vi "LAOnMessage.vi"(8 "Error In":errorcluster, 11 "LiteAgent In":T2) -> (0 "Error Out":errorcluster, 1 "AgentMessage":T1, 2 "SessionId":string, 3 "LiteAgent Out":T2)   [LabVIEW 2017, in "LiteAgentSDK.lvlib"]
uses:
  LiteAgentSDK.lvlib
  C:/Users/Jan/Projects/LiteAgentSDK-LabVIEW/Source/Bin/LiteAgentSDK.LabVIEW.dll
  Bin/LiteAgentSDK.LabVIEW.dll
  <vilib>/LVH/i3 JSON/JSON Parsing/Get Object Parameter Files/Get Object Parameter - String.vi
  <vilib>/LVH/i3 JSON/JSON Parsing/Get Object Parameter Files/Get Object Parameter - Object.vi
  <vilib>/LVH/i3 JSON/i3-json.lvlib
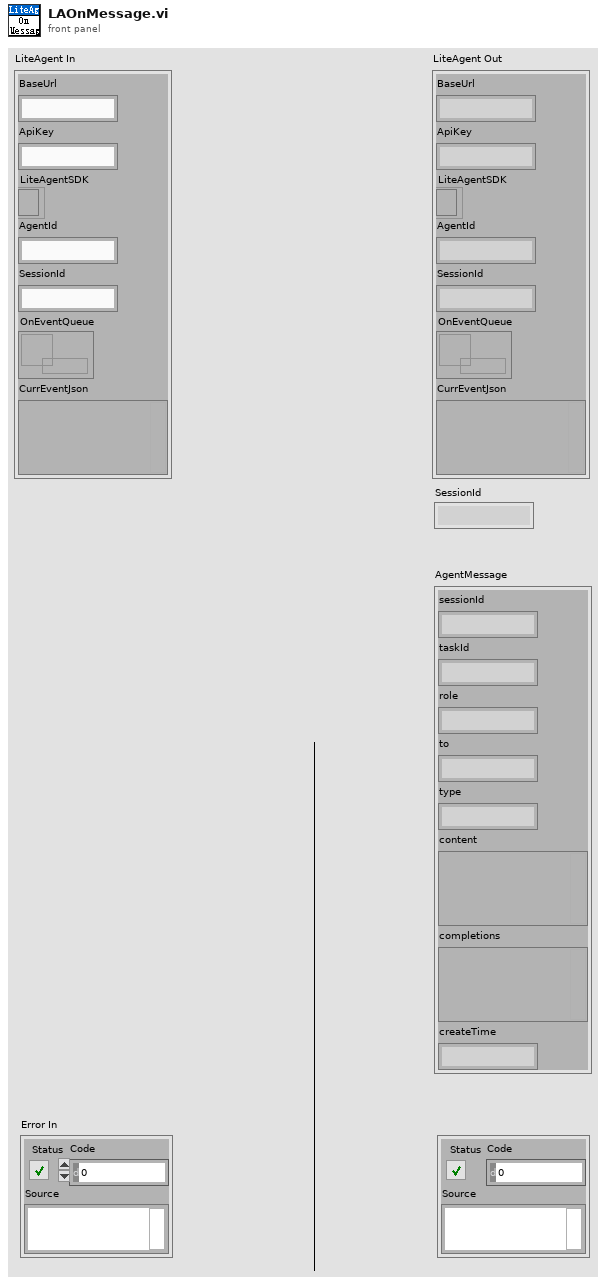
[diagram p1: front panel]
types:
  T1 = cluster{"sessionId":string, "taskId":string, "role":string, "to":string, "type":string, "content":variant, "completions":variant, "createTime":string}
  T2 = cluster{"BaseUrl":string, "ApiKey":string, "LiteAgentSDK":refnum<k24>, "AgentId":string, "SessionId":string, "OnEventQueue":refnum<queue>, "CurrEventJson":variant}
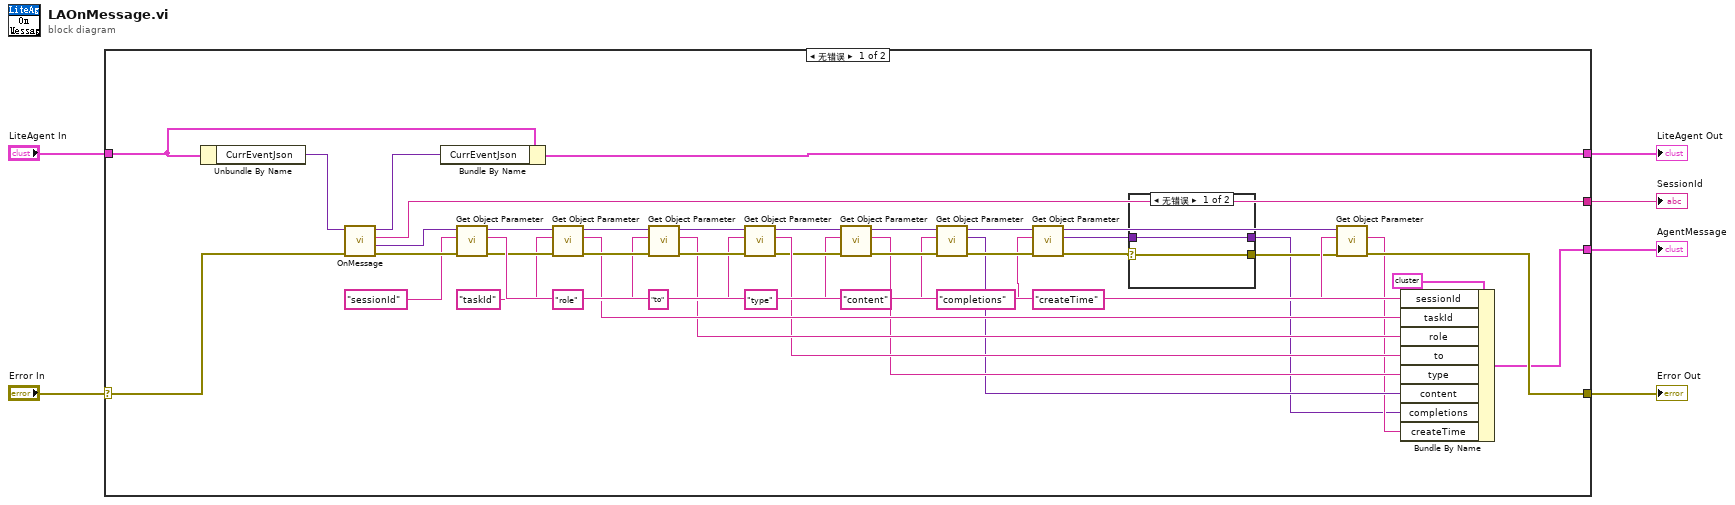
[diagram p0: block diagram]
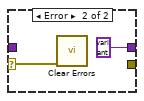
[diagram p2: hidden frame]
diagram:
  n1 = case shown="无错误" "Error In" {
    selector: "Error In" -> [w49 w55]
    tunnel: [w19 w55] -> w5
    tunnel: "LiteAgent In" -> [w47 w54]
    tunnel: [w45 w54] -> w3
    tunnel: [w44 _] -> w2
    tunnel: [w11 _] -> w1
    frame No Error {
      n2 = Unbundle By Name(w47) -> ("CurrEventJson"=w48:variant)
      n3 = call "OnMessage.vi"("Error In"=w49, "JSON Tree In"=w48) -> ("Error Out"=w41:errorcluster, "Payload"=w42:variant, "SessionId"=w44:string, "JSON Tree Out"=w46:variant)  [unwired: 6 in]
      n4 = Bundle By Name(cluster=w47, "CurrEventJson"=w46) -> (w45:T2)
      n5 = call-poly <vilib>:"Get Object Parameter.vi"("error in (no error)"=w41, "Parameter Name"="sessionId", "JSON Tree In (JSON Object)"=w42) -> ("error out"=w37:errorcluster, "String Value"=w39:string, "JSON Tree Out Passthrough"=w38:variant)  [unwired: 5 in, 1 out]
      n6 = call-poly <vilib>:"Get Object Parameter.vi"("error in (no error)"=w37, "Parameter Name"="taskId", "JSON Tree In (JSON Object)"=w38) -> ("error out"=w34:errorcluster, "String Value"=w29:string, "JSON Tree Out Passthrough"=w36:variant)  [unwired: 5 in, 1 out]
      n7 = call-poly <vilib>:"Get Object Parameter.vi"("error in (no error)"=w34, "Parameter Name"="role", "JSON Tree In (JSON Object)"=w36) -> ("error out"=w33:errorcluster, "String Value"=w28:string, "JSON Tree Out Passthrough"=w35:variant)  [unwired: 5 in, 1 out]
      n8 = call-poly <vilib>:"Get Object Parameter.vi"("error in (no error)"=w33, "Parameter Name"="to", "JSON Tree In (JSON Object)"=w35) -> ("error out"=w22:errorcluster, "String Value"=w27:string, "JSON Tree Out Passthrough"=w26:variant)  [unwired: 5 in, 1 out]
      n9 = call-poly <vilib>:"Get Object Parameter.vi"("error in (no error)"=w22, "Parameter Name"="type", "JSON Tree In (JSON Object)"=w26) -> ("error out"=w21:errorcluster, "String Value"=w14:string, "JSON Tree Out Passthrough"=w25:variant)  [unwired: 5 in, 1 out]
      n10 = call-poly <vilib>:"Get Object Parameter.vi"("error in (no error)"=w21, "Parameter Name"="content", "JSON Tree In (JSON Object)"=w25) -> ("error out"=w20:errorcluster, "JSON Object"=w13:variant, "JSON Tree Out Passthrough"=w24:variant)  [unwired: 5 in, 1 out]
      n11 = call-poly <vilib>:"Get Object Parameter.vi"("error in (no error)"=w20, "Parameter Name"="completions", "JSON Tree In (JSON Object)"=w24) -> ("error out"=w10:errorcluster, "JSON Object"=w8:variant, "JSON Tree Out Passthrough"=w23:variant)  [unwired: 5 in, 1 out]
      n12 = case shown="无错误" w10 {
        selector: w10 -> [w51 w53]
        tunnel: [w51 _] -> w9
        tunnel: w8 -> [w50 _]
        tunnel: [w50 variant ("JSON Object")] -> w7
        frame No Error {
        }
        frame Error {
          n13 = call <vilib>:"Clear Errors.vi"("error in (no error)"=w53) -> ()  [unwired: 5 in, 2 out]
        }
      }
      n14 = call-poly <vilib>:"Get Object Parameter.vi"("error in (no error)"=w9, "Parameter Name"="createTime", "JSON Tree In (JSON Object)"=w23) -> ("error out"=w19:errorcluster, "String Value"=w12:string)  [unwired: 5 in, 2 out]
      n15 = Bundle By Name(cluster=T1 {"sessionId"="", "taskId"="", "role"="", "to"="", "type"="", "content"=variant, "completions"=variant, "createTime"=""} ("AgentMessage"), "sessionId"=w39, "taskId"=w29, "role"=w28, "to"=w27, "type"=w14, "content"=w13, "completions"=w7, "createTime"=w12) -> (w11:T1)
    }
    frame Error {
    }
  }
  "Error Out" <- w5
  "LiteAgent Out" <- w3
  "SessionId" <- w2
  "AgentMessage" <- w1
